vi "Create_Error_String_Sub_VI.vi"(8 "error in":errorcluster) -> (0 "error out":errorcluster, 2 "Error String":string)   [LabVIEW 2017]
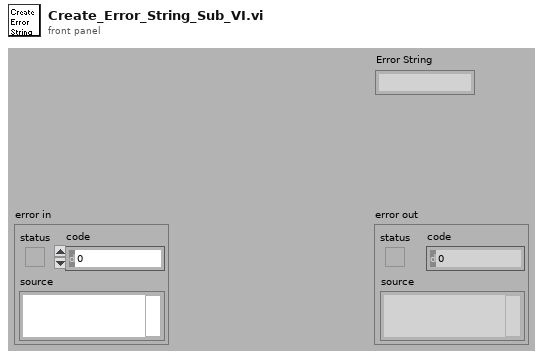
[diagram p1: front panel]
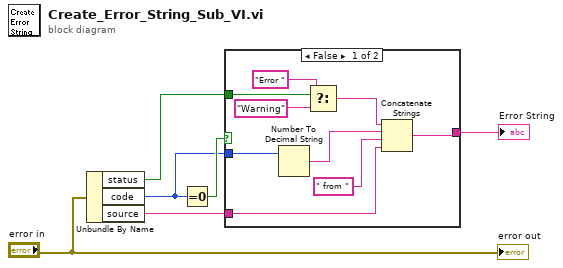
[diagram p0: block diagram]
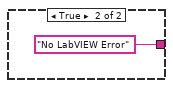
[diagram p2: hidden frame]
diagram:
  n1 = Unbundle By Name("error in") -> ("status"=w3:bool, "code"=w2:i32, "source"=w1:string)
  n2 = Equal To 0?(x=w2) -> (x = 0?=w4:bool)
  n3 = case shown="False" w4 {
    tunnel: [w7 "No LabVIEW Error"] -> w5
    tunnel: w3 -> [w15 _]
    tunnel: w2 -> [w12 _]
    tunnel: w1 -> [w8 _]
    frame False {
      n4 = Number To Decimal String(number=w12) -> (decimal integer string=w10:string)  [unwired: 1 out]
      n5 = Select(t="Error ", s=w15, f="Warning") -> (s? t:f=w11:string)
      n6 = Concatenate Strings(w11, w10, " from " ("string"), w8) -> (w7:string)
    }
    frame True {
    }
  }
  "Error String" <- w5
  "error out" <- "error in"
